vi "NMEA气象仪数据插入.vi"(0 "Tabe Name":string, 1 "data":T1, 2 "Password":string, 3 "错误输入（无错误）":errorcluster, 4 "数据库类型":T2) -> (10 "错误输出":errorcluster)   [LabVIEW 2016]
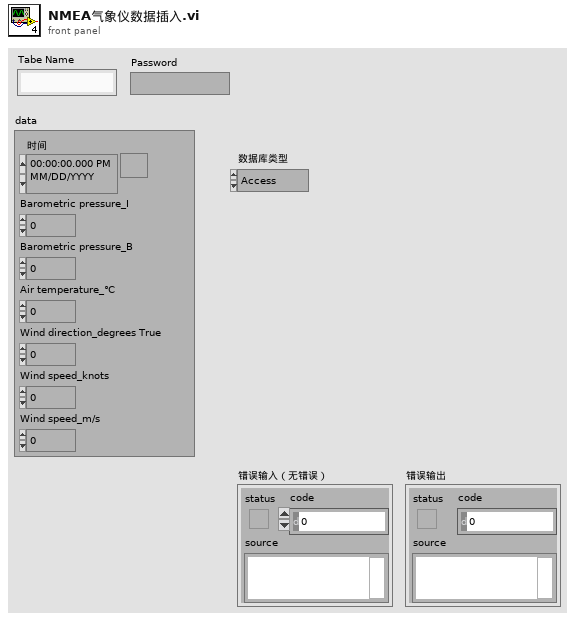
[diagram p1: front panel]
types:
  T1 = typedef "NMAE气象仪字段定义.ctl" = cluster{"时间":timestamp, "Barometric pressure_I":dbl, "Barometric pressure_B":dbl, "Air temperature_℃":dbl, "Wind direction_degrees True":dbl, "Wind speed_knots":dbl, "Wind speed_m/s":dbl}
  T2 = typedef "数据库类型.ctl" = enum16{"Access", "SQLite"}
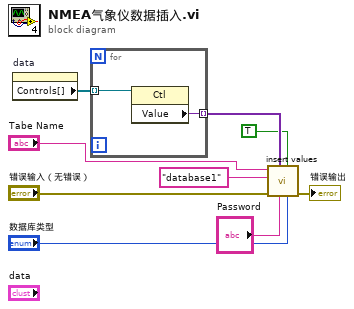
[diagram p0: block diagram]
diagram:
  n1 = property on="data" class="Clust (严格)"() -> ("Controls[]"=w2:refnum<vi>[])  [unwired: 2 in, 2 out]
  n2 = for {
    tunnel: w2 -> [w11] mode=indexing
    tunnel: [w10] -> w9 mode=indexing
    n3 = property class="Ctl"(reference=w11) -> ("Value"=w10:variant)  [unwired: 1 in, 2 out]
  }
  n4 = call "insert values.vi"("数据库类型"="数据库类型", "是否创建唯一键"=TRUE, "Password"="Password", "data"=w9, "错误输入（无错误）"="错误输入（无错误）", "database"="database1", "Tabe Name"="Tabe Name") -> ("错误输出"=→"错误输出":errorcluster)  [unwired: 4 in]
